vi "estruct_case.vi"() -> ()   [LabVIEW 2020]
panel:
  out "Boolean 2":bool
  out "String":string
  in  "Boolean":bool
  in  "stop":bool
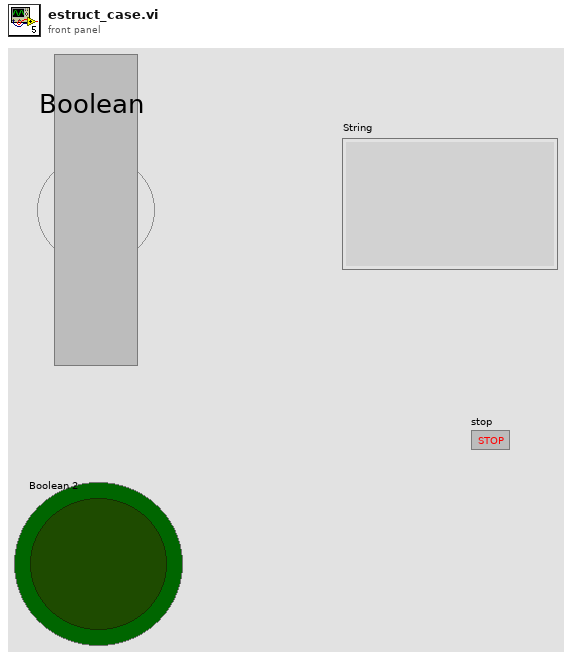
[diagram p1: front panel]
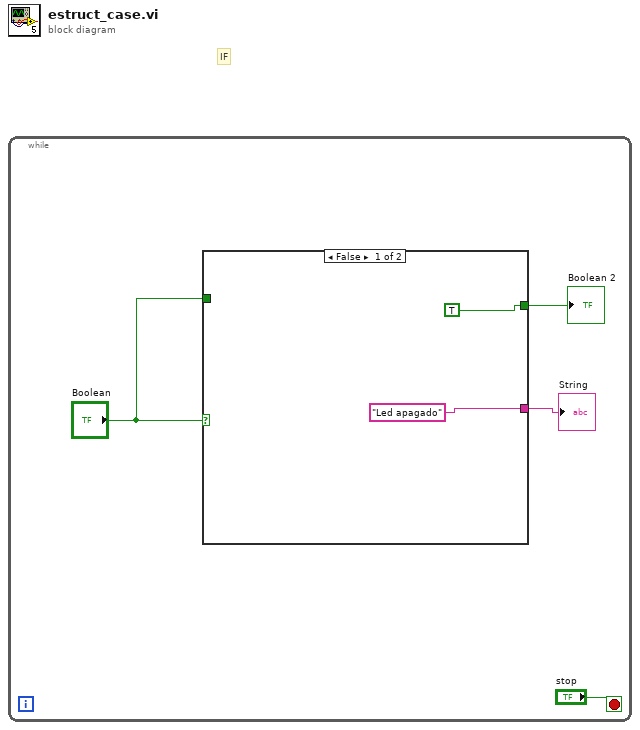
[diagram p0: block diagram]
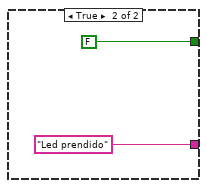
[diagram p2: hidden frame]
diagram:
  # "IF"
  n1 = while {
    stop <- "stop" stop-if-true
    n2 = case shown="False" "Boolean" {
      tunnel: ["Led apagado" "Led prendido"] -> w3
      tunnel: "Boolean" -> [_ _]
      tunnel: [TRUE FALSE] -> w1
      frame False {
      }
      frame True {
      }
    }
    "String" <- w3
    "Boolean 2" <- w1
  }
